vi "cl_serv_cl3.vi"() -> ()   [LabVIEW 2015]
doc: "Establishes a connection to TCP Multiple Connections - Server.vi. After you click the Stop button, this VI sends a single character to tell the Server VI to terminate the connection."
panel:
  out "String":string
  in  "Server Closed 1":string="The server VI closed the connection."
  out "Slide ind":u8(slide) scale=0.0..10.0
  in  "close":bool
  in  "stop":bool
  in  "Connect":bool
  in  "Server Closed":string="The server VI closed the connection."
  in  "Slide ctrl":dbl(slide) scale=0.0..10.0
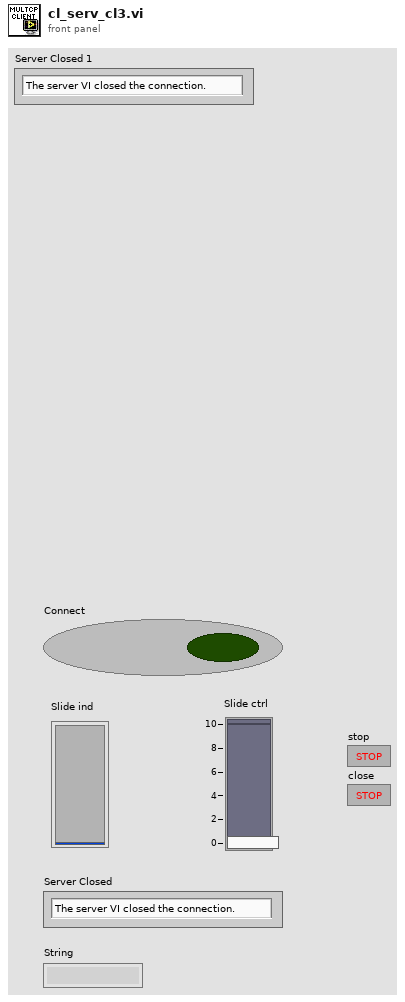
[diagram p1: front panel]
types:
  T1 = enum8{"Enabled", "Disabled", "Disabled and Grayed Out"}
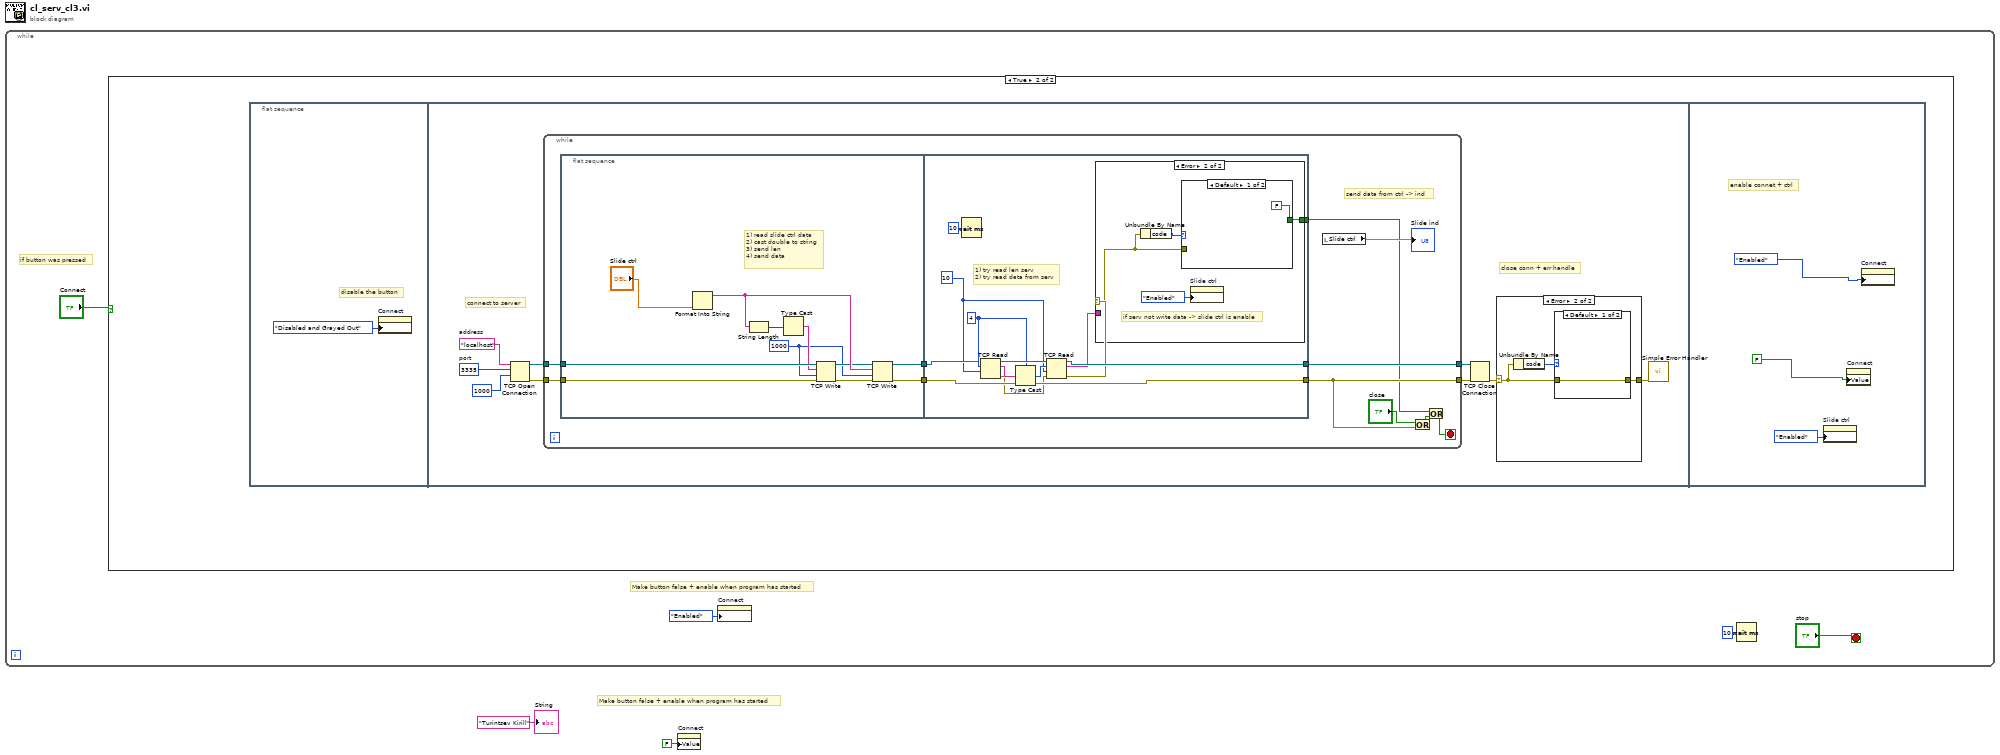
[diagram p0: block diagram]
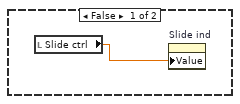
[diagram p2: hidden frame]
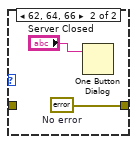
[diagram p4: hidden frame]
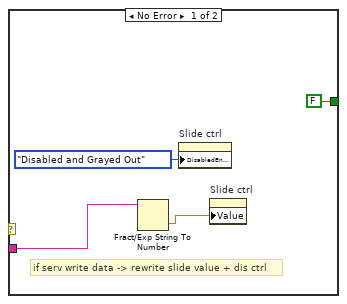
[diagram p5: hidden frame]
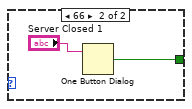
[diagram p6: hidden frame]
diagram:
  # "Make button false + enable when program has started"
  n1 = while {
    stop <- "stop" stop-if-true
    # "Make button false + enable when program has started"
    # "if button was pressed"
    n2 = case shown="True" "Connect" {
      frame False {
        n3 = local read "Slide ctrl"() -> (w7:dbl)
        n4 = property on="Slide ind" class="Slide (strict)"("Value"=w7) -> ()  [unwired: 2 in, 2 out]
      }
      frame True {
        n5 = flat-sequence {
          frame #0 {
            # "disable the button"
            n6 = property on="Connect" class="Bool (strict)"("DisabledEnum"=T1."Disabled and Grayed Out" ("Disabled")) -> ()  [unwired: 2 in, 2 out]
          }
          frame #1 {
            w16 = u16 3335  # port
            w17 = "localhost"  # address
            # "close conn + err handle"
            # "connect to server"
            n7 = TCP Open Connection(address=w17, remote port or service name=w16, timeout ms (60000)=1000) -> (connection ID=w15:refnum<k5>, error out=w14:errorcluster)  [unwired: 1 in, 1 out]
            n8 = while {
              tunnel: [w34] -> w11
              tunnel: [w35] -> w10
              tunnel: w14 -> [w32]
              tunnel: w15 -> [w33]
              stop <- w27 stop-if-true
              # "send data from ctrl -> ind"
              n9 = flat-sequence {
                tunnel: w33 -> [w42]
                tunnel: w32 -> [w40]
                tunnel: [w46] -> w31
                tunnel: [w45] -> w30
                tunnel: [w52] -> w34
                tunnel: [w58] -> w35
                tunnel: w31 -> [w58]
                tunnel: w30 -> [w53]
                tunnel: [w47] -> w25
                frame #0 {
                  w36 = 1000 ("timeout ms (25000)")
                  # "1) read slide ctrl data\n2) cast double to string\n3) send len\n4) send data"
                  n10 = Format Into String("Slide ctrl") -> (resulting string=w43:string)  [unwired: 3 in, 1 out]
                  n11 = String Length(string=w43) -> (length=w38:i32)
                  n12 = Type Cast(x=w38) -> (*(type *) &x=w37:string)  [unwired: 1 out]
                  n13 = TCP Write(connection ID=w42, data in=w37, error in (no error)=w40, 9:w36) -> (connection ID out=w41:refnum<k5>, error out=w39:errorcluster)  [unwired: 1 out]
                  n14 = TCP Write(connection ID=w41, data in=w43, error in (no error)=w39, 9:w36) -> (connection ID out=w45:refnum<k5>, error out=w46:errorcluster)  [unwired: 1 out]
                }
                frame #1 {
                  w51 = 10 ("timeout ms (25000)")
                  w54 = 4 ("bytes to read")
                  # "1) try read len serv\n2) try read data from serv"
                  n15 = Wait (ms)(milliseconds to wait=u32 10) -> ()  [unwired: 1 out]
                  n16 = TCP Read(connection ID=w53, bytes to read=w54, 9:w51) -> (connection ID out=w57:refnum<k5>, data out=w56:string, error out=w48:errorcluster)  [unwired: 2 in]
                  n17 = Type Cast(type=w54, x=w56) -> (*(type *) &x=w55:i32)
                  n18 = TCP Read(connection ID=w57, bytes to read=w55, error in (no error)=w48, 9:w51) -> (connection ID out=w52:refnum<k5>, data out=w50:string, error out=w49:errorcluster)  [unwired: 1 in]
                  n19 = case shown="Error" w49 {
                    selector: w49 -> [_ w66]
                    tunnel: w50 -> [w63 _]
                    tunnel: [FALSE ("true") w65] -> w47
                    frame No Error {
                      # "if serv write data -> rewrite slide value + dis ctrl"
                      n20 = Fract/Exp String To Number(string=w63) -> (number=w62:dbl)  [unwired: 3 in, 1 out]
                      n21 = property on="Slide ctrl" class="Slide (strict)"("DisabledEnum"=T1."Disabled and Grayed Out" ("Disabled")) -> ()  [unwired: 2 in, 2 out]
                      n22 = property on="Slide ctrl" class="Slide (strict)"("Value"=w62) -> ()  [unwired: 2 in, 2 out]
                    }
                    frame Error {
                      # "if serv not write data -> slide ctrl is enable"
                      n23 = Unbundle By Name(w66) -> ("code"=w67:i32)
                      n24 = case shown="Default" w67 {
                        tunnel: w66 -> [_ _]
                        tunnel: [FALSE ("true") w69] -> w65
                        frame Default {
                        }
                        frame 66 {
                          n25 = One Button Dialog(message="Server Closed 1") -> (true=w69:bool)  [unwired: 1 in]
                        }
                      }
                      n26 = property on="Slide ctrl" class="Slide (strict)"("DisabledEnum"=T1."Enabled" ("Disabled")) -> ()  [unwired: 2 in, 2 out]
                    }
                  }
                }
              }
              n27 = local read "Slide ctrl"() -> (→"Slide ind":dbl)
              n28 = Or(x="close", y=w35) -> (x .or. y?=w26:bool)
              n29 = Or(x=w25, y=w26) -> (x .or. y?=w27:bool)
            }
            n30 = TCP Close Connection(connection ID=w11, error in (no error)=w10) -> (error out=w13:errorcluster)  [unwired: 2 out]
            n31 = case shown="Error" w13 {
              selector: w13 -> [w18 w20]
              tunnel: [w18 w19] -> w12
              frame No Error {
              }
              frame Error {
                n32 = Unbundle By Name(w20) -> ("code"=w21:i32)
                n33 = case shown="Default" w21 {
                  tunnel: w20 -> [w22 _]
                  tunnel: [w22 w24] -> w19
                  frame Default {
                  }
                  frame 62, 64, 66 {
                    w24 = errorcluster {"status"=FALSE, "code"=0, "source"=""}  # No error
                    n34 = One Button Dialog(message="Server Closed") -> ()  [unwired: 1 in, 1 out]
                  }
                }
              }
            }
            n35 = call <vilib>:"Simple Error Handler.vi"("error in (no error)"=w12) -> ()  [unwired: 1 in, 8 out]
          }
          frame #2 {
            # "enable connet + ctrl"
            n36 = property on="Slide ctrl" class="Slide (strict)"("DisabledEnum"=T1."Enabled" ("Disabled")) -> ()  [unwired: 2 in, 2 out]
            n37 = property on="Connect" class="Bool (strict)"("Value"=FALSE ("Connect")) -> ()  [unwired: 2 in, 2 out]
            n38 = property on="Connect" class="Bool (strict)"("DisabledEnum"=T1."Enabled" ("Disabled")) -> ()  [unwired: 2 in, 2 out]
          }
        }
      }
    }
    n39 = property on="Connect" class="Bool (strict)"("DisabledEnum"=T1."Enabled" ("Disabled")) -> ()  [unwired: 2 in, 2 out]
    n40 = Wait (ms)(milliseconds to wait=u32 10) -> ()  [unwired: 1 out]
  }
  n41 = property on="Connect" class="Bool (strict)"("Value"=FALSE ("Connect")) -> ()  [unwired: 2 in, 2 out]
  "String" <- "Turintsev Kirill" ("String")
